vi "Read First call.vi"(8 "error in (no error)":errorcluster, 11 "Timer in":refnum<class "Timer.lvclass">) -> (0 "error out":errorcluster, 2 "First call":bool, 3 "Timer out":refnum<class "Timer.lvclass">)   [LabVIEW 2016, in "Timer.lvclass"]
uses:
  Timer.lvclass
  Timer.lvclass/Timer.ctl
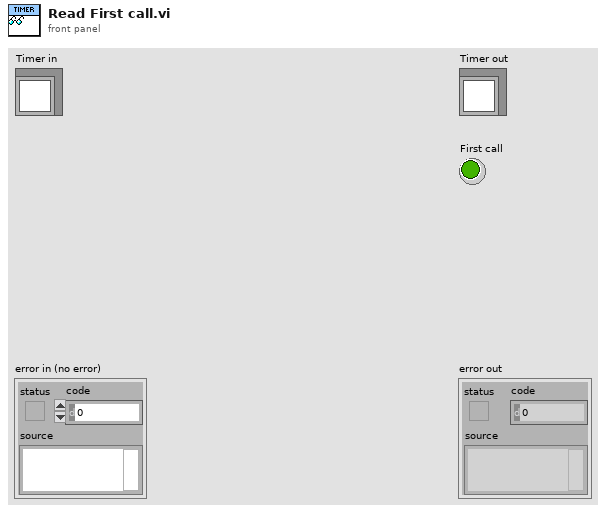
[diagram p1: front panel]
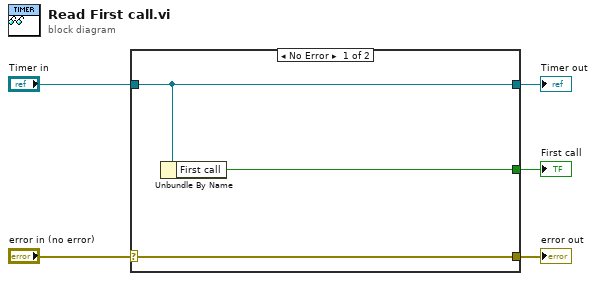
[diagram p0: block diagram]
diagram:
  n1 = case shown="No Error" "error in (no error)" {
    selector: "error in (no error)" -> [w8 w9]
    tunnel: [w8 w9] -> w4
    tunnel: [w7 w10] -> w2
    tunnel: "Timer in" -> [w7 w10]
    tunnel: [w6 _] -> w1
    frame No Error {
      n2 = Unbundle By Name(w7) -> ("First call"=w6:bool)
    }
    frame Error {
    }
  }
  "error out" <- w4
  "Timer out" <- w2
  "First call" <- w1
